vi "SafeMove.vi"(7 "Calibration Constant":dbl, 9 "Axis#":i16 min=0 max=2 step=1, 10 "Forward/Reverse":bool, 11 "Total Distance (mm)":dbl) -> (8 "5V Indicator":bool)   [LabVIEW 2017]
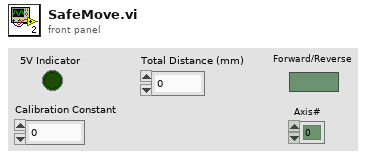
[diagram p1: front panel]
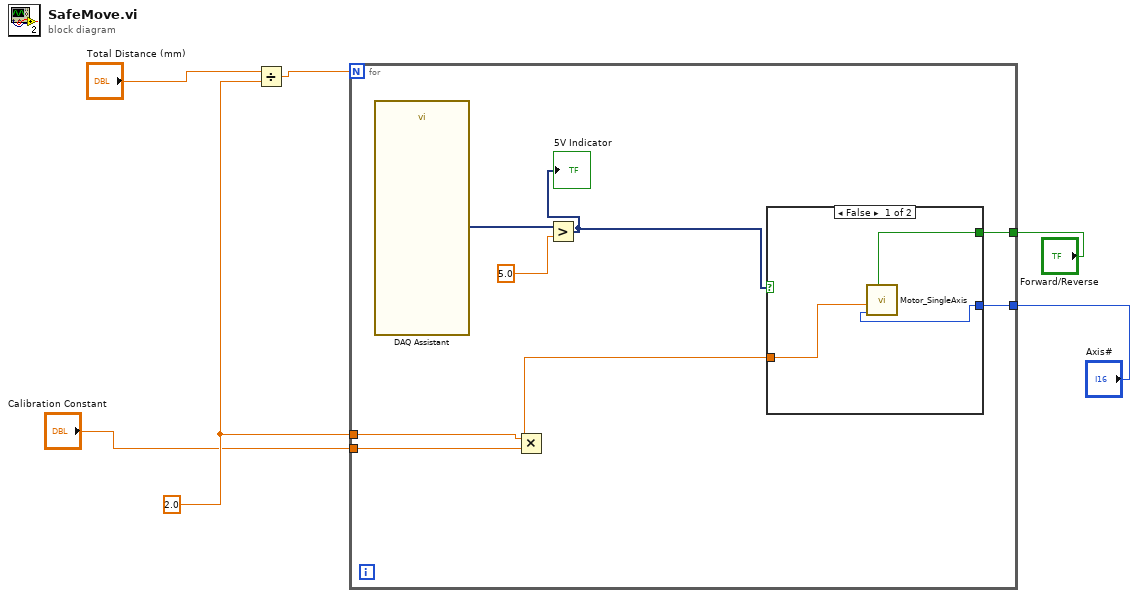
[diagram p0: block diagram]
diagram:
  w4 = 2.0 ("y")
  n1 = Divide(x="Total Distance (mm)", y=w4) -> (x/y=w6:dbl)
  n2 = for {
    N: w6 -> [_]
    tunnel: w4 -> [w10]
    tunnel: "Forward/Reverse" -> [w9]
    tunnel: "Axis#" -> [w8]
    tunnel: "Calibration Constant" -> [w7]
    n3 = call "DAQ Assistant"() -> ("data"=w13:dynamicdata)  [unwired: 17 in, 2 out]
    n4 = Multiply(x=w10, y=w7) -> (x*y=w12:dbl)
    n5 = Greater?(x=w13, y=5.0) -> (0:w11:dynamicdata)
    "5V Indicator" <- w11
    n6 = case shown="False" w11 {
      tunnel: w12 -> [w15 _]
      tunnel: w9 -> [w17 _]
      tunnel: w8 -> [w16 _]
      frame False {
        n7 = call <userlib>:"Motor_SingleAxis.vi"("# of Steps (x100)"=w15, "Axis#"=w16, "Forward/Reverse"=w17) -> ()  [unwired: 2 in, 2 out]
      }
      frame True {
      }
    }
  }
